vi "extract speedlines.vi"(11 "speedlineFileData":dbl[][](array[numeric])) -> (1 "speedlineID":dbl, 3 "speedlines":cluster{dbl[], dbl[]}[](array[cluster]))   [LabVIEW 2018]
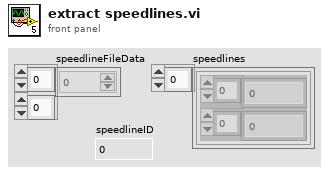
[diagram p1: front panel]
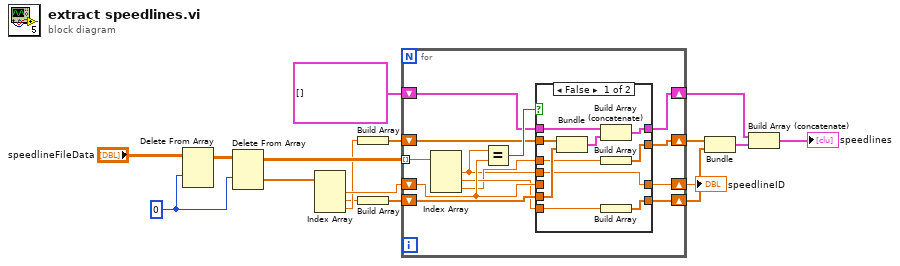
[diagram p0: block diagram]
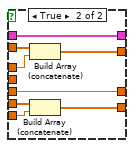
[diagram p2: hidden frame]
diagram:
  w4 = 0 ("index (row)")
  n1 = Delete From Array(array="speedlineFileData", index (row)=w4) -> (array with subset deleted=w3:dbl[][])  [unwired: 2 in, 1 out]
  n2 = Delete From Array(array=w3, index (row)=w4) -> (deleted portion=w5:dbl[], array with subset deleted=w13:dbl[][])  [unwired: 2 in]
  n3 = Index Array(array=w5) -> (element #1=w10:dbl, element #2=w6:dbl, element #3=w7:dbl)  [unwired: 3 in]
  n4 = Build Array(w7) -> (w9:dbl[])
  n5 = Build Array(w6) -> (w8:dbl[])
  n6 = for {
    tunnel: w13 -> [w30] mode=indexing
    shift-right: [w26] -> w15
    shift-left: w8 -> [w25]
    shift-right: [w24] -> w14
    shift-left: w9 -> [w23]
    shift-right: [w28] -> w1
    shift-left: w10 -> [w27]
    shift-right: [w20] -> w12
    shift-left: cluster{dbl[], dbl[]}[] [] -> [w19]
    n7 = Index Array(array=w30) -> (element #1=w18:dbl, element #2=w22:dbl, element #3=w21:dbl)  [unwired: 3 in]
    n8 = Equal?(x=w18, y=w27) -> (x = y?=w29:bool)
    n9 = case shown="False" w29 {
      tunnel: [w35 w48] -> w28
      tunnel: w27 -> [_ w48]
      tunnel: [w33 w45] -> w26
      tunnel: w25 -> [w39 w47]
      tunnel: [w32 w43] -> w24
      tunnel: w23 -> [w40 w46]
      tunnel: w22 -> [w34 w44]
      tunnel: w21 -> [w31 w42]
      tunnel: [w37 w41] -> w20
      tunnel: w19 -> [w38 w41]
      tunnel: w18 -> [w35 _]
      frame False {
        n10 = Bundle(w40, w39) -> (w36:cluster{dbl[], dbl[]})  [unwired: 1 in]
        n11 = Build Array (concatenate)(w38, w36) -> (w37:cluster{dbl[], dbl[]}[])
        n12 = Build Array(w31) -> (w32:dbl[])
        n13 = Build Array(w34) -> (w33:dbl[])
      }
      frame True {
        n14 = Build Array (concatenate)(w46, w42) -> (w43:dbl[])
        n15 = Build Array (concatenate)(w47, w44) -> (w45:dbl[])
      }
    }
  }
  "speedlineID" <- w1
  n16 = Bundle(w14, w15) -> (w16:cluster{dbl[], dbl[]})  [unwired: 1 in]
  n17 = Build Array (concatenate)(w12, w16) -> (→"speedlines":cluster{dbl[], dbl[]}[])
